vi "GV-LightenLineColor_boolean.vi"(2 "Line color":u32(colorbox)) -> (5 "Bool border":u32(colorbox), 6 "Bool envelope":u32(colorbox))   [LabVIEW 2020, in "Sgraph_lib_V1.lvlib" / "Gviewer.lvclass"]
doc: "Andre Koelewijn, 30 june 2021\n\nLighten color for background min/max indication\n26-7-2022 : boolean version (to light teints)"
uses:
  Gviewer.lvclass
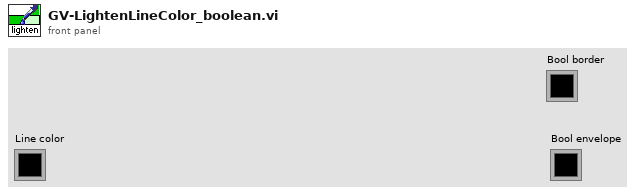
[diagram p1: front panel]
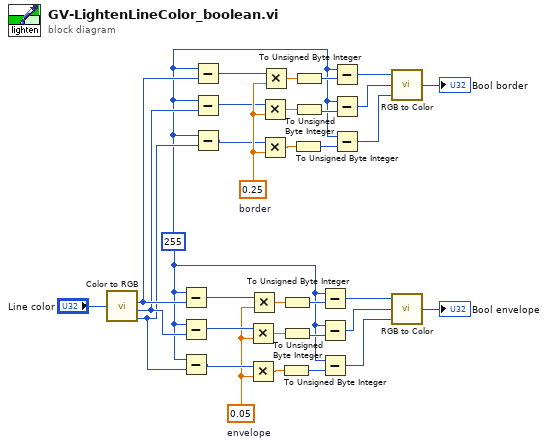
[diagram p0: block diagram]
diagram:
  w12 = 0.25  # border
  w5 = u8 255 ("min/max background")
  w30 = 0.05  # envelope
  n1 = call <vilib>:"Color to RGB.vi"("Color"="Line color") -> ("R"=w8:u8, "G"=w7:u8, "B"=w6:u8)  [unwired: 1 out]
  n2 = Subtract(x=w5, y=w8) -> (x-y=w31:u8)
  n3 = Subtract(x=w5, y=w7) -> (x-y=w32:u8)
  n4 = Subtract(x=w5, y=w6) -> (x-y=w33:u8)
  n5 = Subtract(x=w5, y=w8) -> (x-y=w11:u8)
  n6 = Subtract(x=w5, y=w7) -> (x-y=w10:u8)
  n7 = Subtract(x=w5, y=w6) -> (x-y=w9:u8)
  n8 = Multiply(x=w32, y=w30) -> (x*y=w28:dbl)
  n9 = Multiply(x=w33, y=w30) -> (x*y=w27:dbl)
  n10 = Multiply(x=w31, y=w30) -> (x*y=w29:dbl)
  n11 = Multiply(x=w10, y=w12) -> (x*y=w14:dbl)
  n12 = Multiply(x=w9, y=w12) -> (x*y=w15:dbl)
  n13 = Multiply(x=w11, y=w12) -> (x*y=w13:dbl)
  n14 = To Unsigned Byte Integer(number=w27) -> (unsigned 8bit integer=w24:u8)
  n15 = To Unsigned Byte Integer(number=w29) -> (unsigned 8bit integer=w26:u8)
  n16 = To Unsigned Byte Integer(number=w28) -> (unsigned 8bit integer=w25:u8)
  n17 = To Unsigned Byte Integer(number=w15) -> (unsigned 8bit integer=w18:u8)
  n18 = To Unsigned Byte Integer(number=w13) -> (unsigned 8bit integer=w16:u8)
  n19 = To Unsigned Byte Integer(number=w14) -> (unsigned 8bit integer=w17:u8)
  n20 = Subtract(x=w5, y=w26) -> (x-y=w23:u8)
  n21 = Subtract(x=w5, y=w25) -> (x-y=w22:u8)
  n22 = Subtract(x=w5, y=w24) -> (x-y=w21:u8)
  n23 = Subtract(x=w5, y=w16) -> (x-y=w4:u8)
  n24 = Subtract(x=w5, y=w17) -> (x-y=w3:u8)
  n25 = Subtract(x=w5, y=w18) -> (x-y=w2:u8)
  n26 = call <vilib>:"RGB to Color.vi"("B"=w2, "G"=w3, "R"=w4) -> ("Color"=→"Bool border":u32)
  n27 = call <vilib>:"RGB to Color.vi"("B"=w21, "G"=w22, "R"=w23) -> ("Color"=→"Bool envelope":u32)
